vi "Global Data.vi"() -> ()   [LabVIEW 2014]
uses:
  BMS Telemetry.ctl
  Vehicle Status/Subsystem Status.ctl
  Vehicle Status/Subsystem Status Severity.ctl
  Vehicle Status/Subsystem Status Message.ctl
  FPGA Telemetry.ctl
  AIR Status.ctl
  Reason for Shutdown.ctl
  Dash LED Status.ctl
  FPGA/SPI v2/ADXL345 Output.ctl
  Shutdown State Machine.lvsc/State.ctl
  CAN/MC/MC Temp 1.ctl
  CAN/MC/MC Temp 2.ctl
  CAN/MC/MC Temp 3.ctl
  CAN/MC/MC Current.ctl
  CAN/MC/MC Voltage.ctl
  CAN/MC/MC State.ctl
  CAN/Inverter States.ctl
  CAN/Inverter Run Modes.ctl
  CAN/VSM States.ctl
  CAN/MC/MC Torque.ctl
  CAN/MC/MC Faults.ctl
  CAN/MC/MC Position.ctl
  MC State Machine.lvsc/State.ctl
  CAN/MC/MC Internal Voltages.ctl
  CAN/MC/MC Flux.ctl
  CAN/MC/MC Mod Index and Flux Weakening.ctl
  Dashboard/DashDriverInputs.ctl
  Lap Statistics.ctl
  Dashboard/SDashLEDs.ctl
  CAN/TX Library/CAN Message Queue.ctl
  CAN/TX Library/CAN Message.ctl
  Shutdown State Machine.lvsc
  MC State Machine.lvsc
panel:
  out "HighPriorityCANQueue":T1
  out "LowPriorityCANQueue":T1
  out "MPowerLimiterCorrection":dbl
  out "SDashLEDs":T2
  out "RS232 Error Out":errorcluster
  in  "MTorqueRequest":dbl
  out "SLapStatistics":T3
  out "rAverageThrottle":dbl
  out "tRequestMCControl":dbl
  out "SDashDriverInputs":T4
  out "bPrechargeFailed":bool
  out "Mod Index & Flux Weakening":T5
  out "CAN Interface":refnum<k20>
  out "MC Flux":T6
  out "MC Internal Voltages":T7
  out "iPhone LF Data":cluster{"Lat":dbl, "Long":dbl, "Speed":dbl}
  out "iPhone HF Data":T8
  out "eMCStateMachine":T9=enum."Disabled"
  out "bNewCANLog":bool
  out "bNewSlowFPGALog":bool
  out "bNewFastFPGALog":bool
  in  "CLogFilePrefix":string
  in  "eReasonForShutdown":T10
  in  "bDisableAIRs":bool
  in  "bDisableMC":bool
  out "bRemoteReturnToPits":bool
  out "MC Position":T11
  out "MC Faults":T12 {"MC RUN" format="%x"; "MC Post" format="%x"}
  out "MC Torque":T13
  out "MC State":T14
  out "MC Voltage":T18
  out "MC Current":T19
  out "MC Temp 3":T20
  out "MC Temp 2":T21
  out "MC Temp 1":T22
  in  "bStopCode":bool
  out "eAIRStatus":T23
  out "eShutdownStateMachine":T24=enum."TSMS Off"
  in  "FPGA Telemetry":T25={"CPU Load"={"Total (%)"=16.524459104265105, "Time Critical (%)"=0.0023081499865067385, "Timed Structures (%)"=0.0005419957749163527, "High (%)"=0.304724766613852, "Above Normal (%)"=6.671544042254672, "Normal (%)"=9.519195244591105, "Background (%)"=0.026144905044047956, "Idle (%)"=83.4755408957349, "ISR (%)"=0.0}, "SVehicleStatus"={"BMS Status"={"eStatusSeverity"=enum."Okay", "NValue"=0.0, "CMessage"=enum."ControllerTemperature", "bNotOK"=FALSE}, "MC Status"={"eStatusSeverity"=enum."Okay", "NValue"=0.0, "CMessage"=enum."ControllerTemperature", "bNotOK"=FALSE}, "Shutdown Status"={"eStatusSeverity"=enum."Return to Pits", "NValue"=0.0, "CMessage"=enum."ControllerTemperature", "bNotOK"=FALSE}, "sbRIO Status"={"eStatusSeverity"=enum."Okay", "NValue"=0.0, "CMessage"=enum."ControllerTemperature", "bNotOK"=FALSE}, "Vehicle Status"={"eStatusSeverity"=enum."Return to Pits", "NValue"=0.0, "CMessage"=enum."ControllerTemperature", "bNotOK"=FALSE}, "Shutdown State"=enum."TSMS Off", "AIR Status"=enum."On", "Remote Return to Pits"=TRUE, "Reason for Shutdown"=enum."Shutdown", "MC State Machine Status"=enum."Disabled"}, "iPhone HF Data"={"gXiPhone"=0.0, "gYiPhone"=0.0, "gZiPhone"=0.0, "nYawXiPhone"=0.0, "nYawYiPhone"=0.0, "nYawZiPhone"=0.0}, "iPhone LF Data"={"nLatiPhone"=0.0, "nLongiPhone"=0.0, "nGPSiPhone"=0.0}, "stop"=TRUE, "VSupplyOffset"=0.3359375, "VsbRIOSupply"=0.3803386688232422, "bFPGALED"=TRUE, "TSBRIO"=0.3482666015625, "rTPS2Unscaled"=0.999969482421875, "rTPS1Unscaled"=0.999969482421875, "bTPSConsistent"=TRUE, "bTPSInRange"=FALSE, "rThrottle"=-11.19873046875, "VTPS2"=0.0, "rTPS2"=1.744140625, "VTPS1"=7.0, "rTPS1"=0.0, "rTPS2Max"=0.27001953125, "rTPS2Min"=0.489990234375, "rTPS1Max"=0.6201171875, "rTPS1Min"=0.41015625, "bCoolantPumpEnable"=FALSE, "bRTDSEnable"=TRUE, "bTSMSInStatus"=FALSE, "bPosAIREnable"=TRUE, "bBMSOK"=FALSE, "bIMDOK"=FALSE, "bBSPDOK"=TRUE, "bSBRIOOK2"=TRUE, "bSBRIOOK1"=TRUE, "bTSMSOutStatus"=TRUE, "eGreenDash"=enum."Off", "eYellowDash"=enum."Off", "eRedDash"=enum."Off", "bMotorControllerEnable"=TRUE, "tCurrentLap"=0, "bNewLap"=TRUE, "tLastLap"=0, "tLapMin"=0, "V5VSupply"=0.0, "bWheelRL"=TRUE, "bWheelRR"=TRUE, "bWheelFR"=FALSE, "bWheelFL"=FALSE, "VBrakePressureR"=0.4820976257324219, "VBrakePressureF"=0.4808177947998047, "bWheelRRStopped"=FALSE, "bWheelRLStopped"=FALSE, "bWheelFRStopped"=FALSE, "bWheelFLStopped"=TRUE, "tWheelRLPeriod"=0, "tWheelRRPeriod"=0, "tWheelFRPeriod"=0, "tWheelFLPeriod"=0, "bBrakeLight"=TRUE, "VShockRR"=0.3793773651123047, "VShockRL"=0.3444976806640625, "VShockFR"=0.3425788879394531, "VShockFL"=0.3892974853515625, "IHighCurrent"=-20.724609375, "ILowCurrent"=4.353515625, "pBrakeR"=0.0, "pBrakeF"=0.0, "bHighCurrentOK"=FALSE, "bLowCurrentOK"=FALSE, "bBrakeROK"=FALSE, "bBrakeFOK"=FALSE, "VSteerWheelMiddle"=0.34827280044555664, "aSteerWheel"=124.90449142456055, "nWheelFL"=0.0, "nWheelFR"=0.0, "nWheelRL"=0.0, "nWheelRR"=0.0, "ADXL345 Output"={"X"=0.0, "Y"=0.0, "Z"=0.0}, "Tire Diameter(m)"=0.0, "vWheelRR"=0.0, "vWheelRL"=0.0, "vWheelFR"=0.0, "vWheelFL"=0.0, "vWheelLowest"=0.0, "vWheelHighest"=0.0, "bAccel"=FALSE, "vAxleF"=0.0, "vCar"=0.0, "sLap"=0.0, "rSlipRL"=0.0, "rSlipRR"=0.0, "rSlipFL"=0.0, "rSlipFR"=0.0, "NLap"=0, "tLapReference"=0, "tFastestLap"=0, "MTorqueRequest"=0.0, "RS232 Error Out"={"status"=FALSE, "code"=0}} {"TSBRIO" format="%.10g"; "CPU Load"."ISR (%)" format="%#.2f"; "CPU Load"."Idle (%)" format="%#.2f"; "CPU Load"."Background (%)" format="%#.2f"; "CPU Load"."Normal (%)" format="%#.2f"; "CPU Load"."Above Normal (%)" format="%#.2f"; "CPU Load"."High (%)" format="%#.2g"; "CPU Load"."Time Critical (%)" format="%#.2g"}
  in  "SVehicleStatus":T26
  in  "SSBRIOStatus":T26
  in  "SShutdownStatus":T26
  in  "SMCStatus":T26
  in  "SBMSStatus":T26
  out "BMS Telemetry":T31={"bBMSIgnition"=FALSE, "bBMSChargerMains"=FALSE, "bBMSFastCharge"=FALSE, "bBMSChargerEnabled"=FALSE, "eBMSCarState"=enum."Off", "eBMSChargingState"=enum."Disconnected", "tBMSChargeStage"=32, "eBMSLastChargeError"=enum."No Error", "NBMSNumCells"=70, "bBMSUnderVProtection"=FALSE, "bBMSOverVProtection"=FALSE, "bBMSOverTProtection"=FALSE, "bBMSLeakageProtection"=FALSE, "bBMSNoCellCommsError"=FALSE, "bBMSLowVReduction"=FALSE, "bBMSHighTReduction"=FALSE, "VCellMin"=3.84, "VCellMax"=4.2, "VCellMean"=4.0600000000000005, "VTotal"=284.33, "TCellMin"=17.0, "TCellMax"=43.0, "TCellMean"=20.0, "VCells"={"[51]"=4.08, "[52]"=4.05, "[53]"=4.1, "[54]"=4.2, "[55]"=0.0, "[56]"=4.109999999999999, "[57]"=4.1, "[58]"=4.1899999999999995, "[59]"=4.109999999999999, "[60]"=4.07, "[61]"=4.1, "[62]"=4.220000000000001, "[63]"=0.0, "[64]"=4.07, "[65]"=4.05, "[66]"=4.109999999999999, "[67]"=4.12, "[34]"=3.95, "[35]"=4.05, "[36]"=4.1, "[37]"=4.08, "[38]"=4.05, "[39]"=0.0, "[40]"=4.07, "[41]"=4.029999999999999, "[42]"=4.02, "[43]"=4.02, "[44]"=3.99, "[45]"=4.05, "[46]"=4.029999999999999, "[47]"=0.0, "[48]"=3.99, "[49]"=4.01, "[50]"=4.02, "[17]"=3.84, "[18]"=4.0600000000000005, "[19]"=4.05, "[20]"=3.99, "[21]"=4.02, "[22]"=4.02, "[23]"=0.0, "[24]"=4.07, "[25]"=4.01, "[26]"=4.140000000000001, "[27]"=4.02, "[28]"=4.05, "[29]"=4.029999999999999, "[30]"=4.08, "[31]"=0.0, "[32]"=4.109999999999999, "[33]"=4.02, "[0]"=2.0, "[1]"=2.0, "[2]"=2.0, "[3]"=2.0, "[4]"=2.0, "[5]"=2.0, "[6]"=2.0, "[7]"=0.0, "[8]"=4.02, "[9]"=4.07, "[10]"=4.029999999999999, "[11]"=4.02, "[12]"=4.02, "[13]"=4.05, "[14]"=4.0600000000000005, "[15]"=0.0, "[16]"=4.2}, "TCells"={"[55]"=0.0, "[56]"=21.0, "[57]"=21.0, "[58]"=33.0, "[59]"=21.0, "[60]"=23.0, "[61]"=21.0, "[62]"=43.0, "[63]"=0.0, "[64]"=22.0, "[65]"=21.0, "[66]"=21.0, "[67]"=19.0, "[68]"=21.0, "[69]"=20.0, "[70]"=-100.0, "[17]"=19.0, "[38]"=21.0, "[39]"=0.0, "[40]"=19.0, "[41]"=21.0, "[42]"=21.0, "[43]"=21.0, "[44]"=19.0, "[45]"=21.0, "[46]"=20.0, "[47]"=0.0, "[48]"=20.0, "[49]"=19.0, "[50]"=19.0, "[51]"=19.0, "[52]"=19.0, "[53]"=19.0, "[54]"=33.0, "[21]"=20.0, "[22]"=20.0, "[23]"=0.0, "[24]"=21.0, "[25]"=21.0, "[26]"=21.0, "[27]"=19.0, "[28]"=19.0, "[29]"=19.0, "[30]"=19.0, "[31]"=0.0, "[32]"=19.0, "[33]"=19.0, "[34]"=19.0, "[35]"=19.0, "[36]"=19.0, "[37]"=19.0, "[0]"=19.0, "[1]"=17.0, "[2]"=19.0, "[3]"=19.0, "[4]"=19.0, "[5]"=19.0, "[6]"=19.0, "[7]"=0.0, "[8]"=21.0, "[9]"=19.0, "[10]"=20.0, "[11]"=19.0, "[12]"=21.0, "[13]"=19.0, "[14]"=19.0, "[15]"=0.0, "[16]"=25.0}, "bChargerConnected"=FALSE, "VChargerSetpoint"=0.0, "IChargerSetpoint"=0.0, "VChargerActual"=0.0, "IChargerActual"=0.0, "BCells"={"[51]"=0.0, "[52]"=0.0, "[53]"=0.0, "[54]"=0.0, "[55]"=0.0, "[56]"=0.0, "[57]"=0.0, "[58]"=0.0, "[59]"=0.0, "[60]"=0.0, "[61]"=0.0, "[62]"=0.0, "[63]"=0.0, "[64]"=0.0, "[65]"=0.0, "[66]"=0.0, "[67]"=0.0, "[34]"=0.0, "[35]"=0.0, "[36]"=0.0, "[37]"=0.0, "[38]"=0.0, "[39]"=0.0, "[40]"=0.0, "[41]"=0.0, "[42]"=0.0, "[43]"=0.0, "[44]"=0.0, "[45]"=0.0, "[46]"=0.0, "[47]"=0.0, "[48]"=0.0, "[49]"=0.0, "[50]"=0.0, "[17]"=0.0, "[18]"=0.0, "[19]"=0.0, "[20]"=0.0, "[21]"=0.0, "[22]"=0.0, "[23]"=0.0, "[24]"=0.0, "[25]"=0.0, "[26]"=0.0, "[27]"=0.0, "[28]"=0.0, "[29]"=0.0, "[30]"=0.0, "[31]"=0.0, "[32]"=0.0, "[33]"=0.0, "[0]"=0.0, "[1]"=0.0, "[2]"=0.0, "[3]"=0.0, "[4]"=0.0, "[5]"=0.0, "[6]"=0.0, "[7]"=0.0, "[8]"=0.0, "[9]"=0.0, "[10]"=0.0, "[11]"=0.0, "[12]"=0.0, "[13]"=0.0, "[14]"=0.0, "[15]"=0.0, "[16]"=0.0}}
  in  "bMCOn":bool
  in  "bEnableRTDS":bool
  in  "nHeading":i16
  in  "nChassis":dbl
  # "MC Telemetry"
  # "Inputs"
  # "Protection"
  # "State"
  # "Outputs"
  # "Reduction"
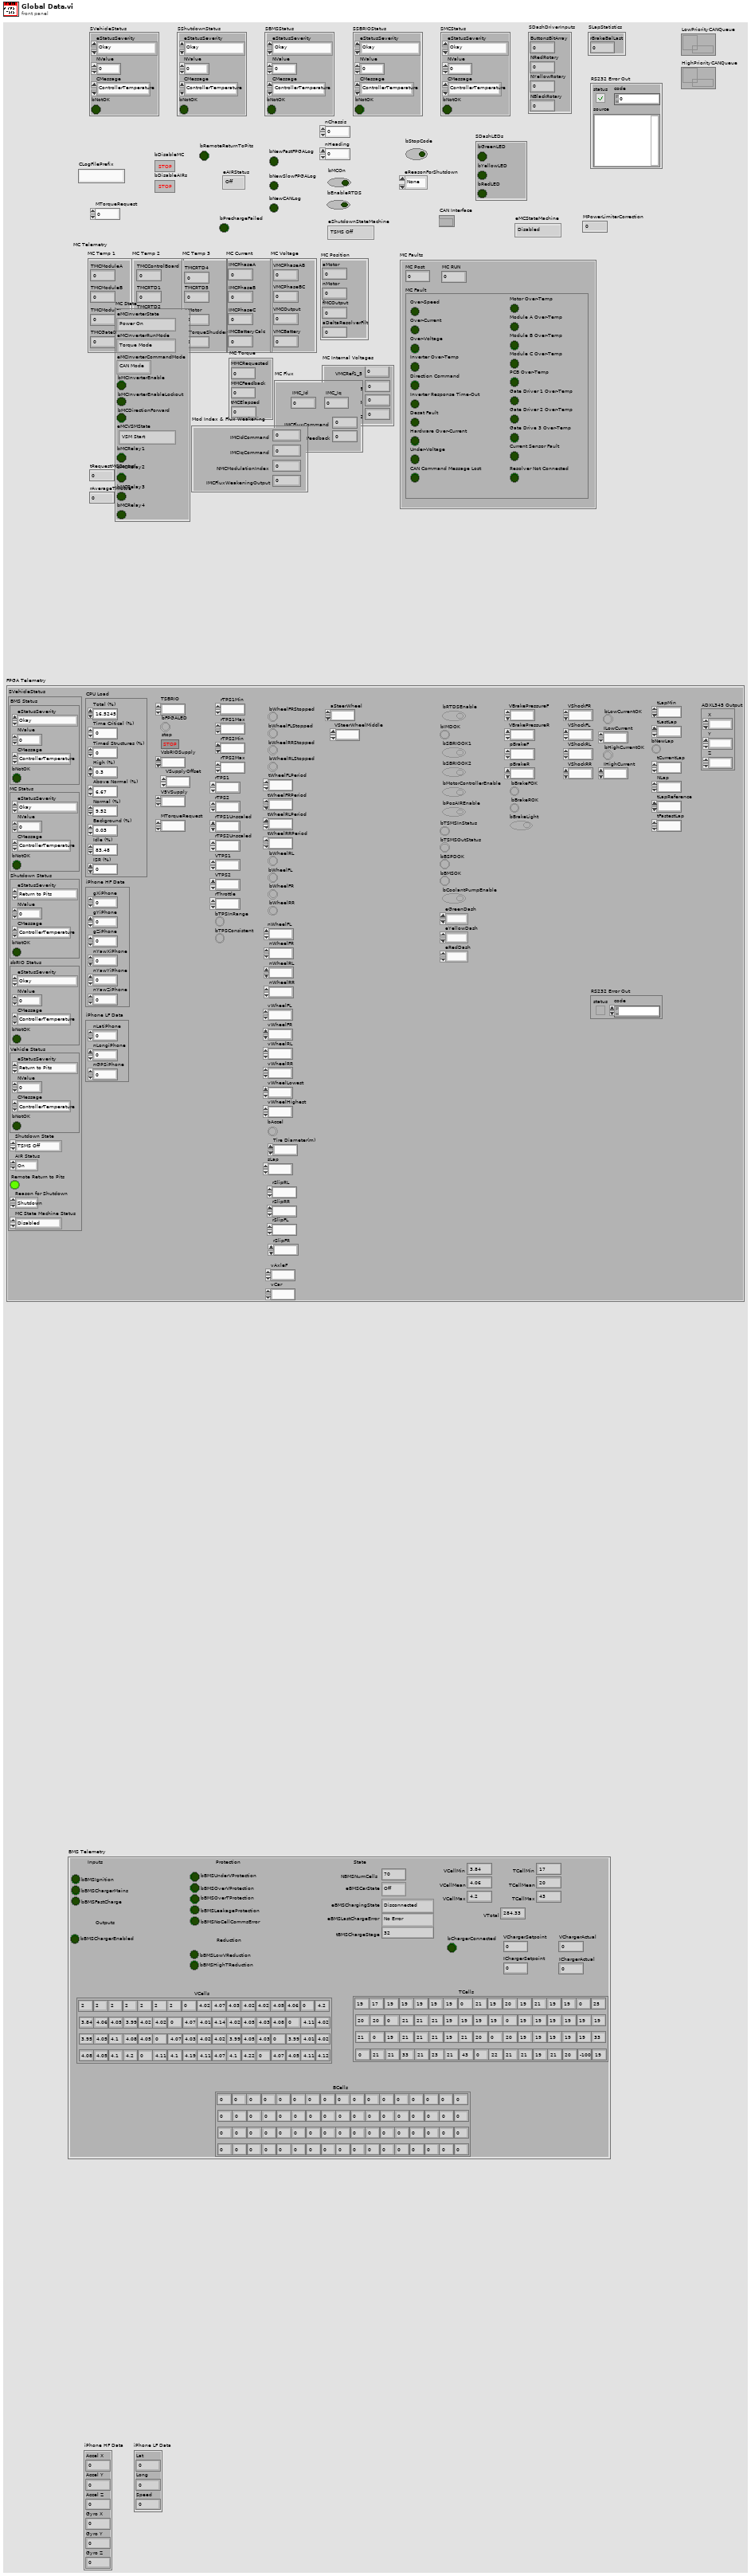
[diagram p1: front panel]
types:
  T1 = typedef "CAN Message Queue.ctl" = refnum<k33>
  T2 = typedef "SDashLEDs.ctl" = cluster{"bGreenLED":bool, "bYellowLED":bool, "bRedLED":bool}
  T3 = typedef "Lap Statistics.ctl" = cluster{"rBrakeBalLast":dbl}
  T4 = typedef "DashDriverInputs.ctl" = cluster{"ButtonsBitArray":u8, "NRedRotary":u8, "NYellowRotary":u8, "NBlackRotary":u8}
  T5 = typedef "MC Mod Index and Flux Weakening.ctl" = cluster{"NMCModulationIndex":dbl, "IMCFluxWeakeningOutput":dbl, "IMCIdCommand":dbl, "IMCIqCommand":dbl}
  T6 = typedef "MC Flux.ctl" = cluster{"IMCFluxCommand":dbl, "IMCFluxFeedback":dbl, "IMC_Id":dbl, "IMC_Iq":dbl}
  T7 = typedef "MC Internal Voltages.ctl" = cluster{"VMCRef1_5":dbl, "VMCRef2_5":dbl, "VMCRef5":dbl, "VMCRef12":dbl}
  T8 = cluster{"Accel X":dbl, "Accel Y":dbl, "Accel Z":dbl, "Gyro X":dbl, "Gyro Y":dbl, "Gyro Z":dbl}
  T9 = typedef "MC State Machine.lvsc/State.ctl" = enum16{"NI.SC.Initial", "NI.SC.History", "NI.SC.ShallowHistory", "NI.SC.Terminal", "Broadcast Diag", "Let Current Drop then Disable AIR's", "Enabled", "Disabled"}
  T10 = typedef "Reason for Shutdown.ctl" = enum16{"None", "BMS", "Shutdown", "sbRIO", "MC", "Remote"}
  T11 = typedef "MC Position.ctl" = cluster{"aMotor":dbl, "nMotor":dbl, "fMCOutput":dbl, "aDeltaResolverFilt":dbl}
  T12 = typedef "MC Faults.ctl" = cluster{"MC Fault":cluster{"Over-Speed":bool, "Over-Current":bool, "Over-Voltage":bool, "Inverter Over-Temp":bool, "Direction Command":bool, "Inverter Response Time-Out":bool, "Desat Fault":bool, "Hardware Over-Current":bool, "Under-Voltage":bool, "CAN Command Message Lost":bool, "Motor Over-Temp":bool, "Module A Over-Temp":bool, "Module B Over-Temp":bool, "Module C Over-Temp":bool, "PCB Over-Temp":bool, "Gate Driver 1 Over-Temp":bool, "Gate Driver 2 Over-Temp":bool, "Gate Drive 3 Over-Temp":bool, "Current Sensor Fault":bool, "Resolver Not Connected":bool}, "MC Post":u32, "MC RUN":u32}
  T13 = typedef "MC Torque.ctl" = cluster{"MMCRequested":dbl, "MMCFeedback":dbl, "tMCElapsed":u32}
  T14 = typedef "MC State.ctl" = cluster{"eMCInverterState":T15, "eMCInverterRunMode":T16, "eMCInverterCommandMode":enum16{"CAN Mode", "VSM Mode"}, "bMCInverterEnable":bool, "bMCInverterEnableLockout":bool, "bMCDirectionForward":bool, "eMCVSMState":T17, "bMCRelay1":bool, "bMCRelay2":bool, "bMCRelay3":bool, "bMCRelay4":bool}
  T15 = typedef "Inverter States.ctl" = enum16{"Power On", "Stop", "Open Loop", "Closed Loop", "Wait", "Internal", "Idle Run", "Idle Stop", ""}
  T16 = typedef "Inverter Run Modes.ctl" = enum16{"Torque Mode", "Speed Mode"}
  T17 = typedef "VSM States.ctl" = enum16{"VSM Start", "Pre-Charge Init", "Pre-Charge Active", "Pre-Charge Complete", "VSM Wait", "VSM Ready", "Motor Running", "Blink Fault Code", "Shutdown in Process", "Recycle Power"}
  T18 = typedef "MC Voltage.ctl" = cluster{"VMCPhaseAB":dbl, "VMCPhaseBC":dbl, "VMCOutput":dbl, "VMCBattery":dbl}
  T19 = typedef "MC Current.ctl" = cluster{"IMCPhaseA":dbl, "IMCPhaseB":dbl, "IMCPhaseC":dbl, "IMCBatteryCalc":dbl}
  T20 = typedef "MC Temp 3.ctl" = cluster{"TMCRTD4":dbl, "TMCRTD5":dbl, "TMotor":dbl, "MTorqueShudder":dbl}
  T21 = typedef "MC Temp 2.ctl" = cluster{"TMCControlBoard":dbl, "TMCRTD1":dbl, "TMCRTD2":dbl, "TMCRTD3":dbl}
  T22 = typedef "MC Temp 1.ctl" = cluster{"TMCModuleA":dbl, "TMCModuleB":dbl, "TMCModuleC":dbl, "TMCGateDriver":dbl}
  T23 = typedef "AIR Status.ctl" = enum16{"Off", "Precharge", "On"}
  T24 = typedef "Shutdown State Machine.lvsc/State.ctl" = enum16{"NI.SC.Initial", "NI.SC.History", "NI.SC.ShallowHistory", "NI.SC.Terminal", "Coolant Pump Started/AIR's On", "AIRs On", "Precharge", "TSMS Off"}
  T25 = typedef "FPGA Telemetry.ctl" = cluster{"CPU Load":cluster{"Total (%)":dbl, "Time Critical (%)":dbl, "Timed Structures (%)":dbl, "High (%)":dbl, "Above Normal (%)":dbl, "Normal (%)":dbl, "Background (%)":dbl, "Idle (%)":dbl, "ISR (%)":dbl}, "SVehicleStatus":cluster{"BMS Status":T26, "MC Status":T26, "Shutdown Status":T26, "sbRIO Status":T26, "Vehicle Status":T26, "Shutdown State":enum16{"NI.SC.Initial", "NI.SC.History", "NI.SC.ShallowHistory", "NI.SC.Terminal", "Coolant Pump Started/AIR's On", "AIRs On", "Precharge", "TSMS Off"}, "AIR Status":T23, "Remote Return to Pits":bool, "Reason for Shutdown":T10, "MC State Machine Status":enum16{"NI.SC.Initial", "NI.SC.History", "NI.SC.ShallowHistory", "NI.SC.Terminal", "Broadcast Diag", "Let Current Drop then Disable AIR's", "Enabled", "Disabled"}}, "iPhone HF Data":cluster{"gXiPhone":dbl, "gYiPhone":dbl, "gZiPhone":dbl, "nYawXiPhone":dbl, "nYawYiPhone":dbl, "nYawZiPhone":dbl}, "iPhone LF Data":cluster{"nLatiPhone":dbl, "nLongiPhone":dbl, "nGPSiPhone":dbl}, "stop":bool, "VSupplyOffset":fxp<+,12,4>, "VsbRIOSupply":fxp<+/-,25,6>, "bFPGALED":bool, "TSBRIO":fxp<+/-,33,17>, "rTPS2Unscaled":fxp<+/-,16,1>, "rTPS1Unscaled":fxp<+/-,16,1>, "bTPSConsistent":bool, "bTPSInRange":bool, "rThrottle":fxp<+/-,33,22>, "VTPS2":fxp<+/-,24,5>, "rTPS2":fxp<+/-,31,22>, "VTPS1":fxp<+/-,24,5>, "rTPS1":fxp<+/-,31,22>, "rTPS2Max":fxp<+,16,4>, "rTPS2Min":fxp<+,16,4>, "rTPS1Max":fxp<+,16,4>, "rTPS1Min":fxp<+,16,4>, "bCoolantPumpEnable":bool, "bRTDSEnable":bool, "bTSMSInStatus":bool, "bPosAIREnable":bool, "bBMSOK":bool, "bIMDOK":bool, "bBSPDOK":bool, "bSBRIOOK2":bool, "bSBRIOOK1":bool, "bTSMSOutStatus":bool, "eGreenDash":T29, "eYellowDash":T29, "eRedDash":T29, "bMotorControllerEnable":bool, "tCurrentLap":u32, "bNewLap":bool, "tLastLap":u32, "tLapMin":u32, "V5VSupply":fxp<+/-,24,5>, "bWheelRL":bool, "bWheelRR":bool, "bWheelFR":bool, "bWheelFL":bool, "VBrakePressureR":fxp<+/-,24,5>, "VBrakePressureF":fxp<+/-,24,5>, "bWheelRRStopped":bool, "bWheelRLStopped":bool, "bWheelFRStopped":bool, "bWheelFLStopped":bool, "tWheelRLPeriod":u32, "tWheelRRPeriod":u32, "tWheelFRPeriod":u32, "tWheelFLPeriod":u32, "bBrakeLight":bool, "VShockRR":fxp<+/-,24,5>, "VShockRL":fxp<+/-,24,5>, "VShockFR":fxp<+/-,24,5>, "VShockFL":fxp<+/-,24,5>, "IHighCurrent":fxp<+/-,24,15>, "ILowCurrent":fxp<+/-,24,15>, "pBrakeR":fxp<+,26,13>, "pBrakeF":fxp<+,26,13>, "bHighCurrentOK":bool, "bLowCurrentOK":bool, "bBrakeROK":bool, "bBrakeFOK":bool, "VSteerWheelMiddle":fxp<+/-,26,5>, "aSteerWheel":fxp<+/-,31,13>, "nWheelFL":fxp<+/-,32,16>, "nWheelFR":fxp<+/-,32,16>, "nWheelRL":fxp<+/-,32,16>, "nWheelRR":fxp<+/-,32,16>, "ADXL345 Output":T30, "Tire Diameter(m)":fxp<+,16,1>, "vWheelRR":fxp<+/-,32,18>, "vWheelRL":fxp<+/-,32,18>, "vWheelFR":fxp<+/-,32,18>, "vWheelFL":fxp<+/-,32,18>, "vWheelLowest":fxp<+/-,32,18>, "vWheelHighest":fxp<+/-,32,18>, "bAccel":bool, "vAxleF":fxp<+/-,33,19>, "vCar":fxp<+/-,33,19>, "sLap":fxp<+,32,12>, "rSlipRL":fxp<+/-,12,1>, "rSlipRR":fxp<+/-,12,1>, "rSlipFL":fxp<+/-,12,1>, "rSlipFR":fxp<+/-,12,1>, "NLap":u8, "tLapReference":u32, "tFastestLap":u32, "MTorqueRequest":dbl, "RS232 Error Out":cluster{"status":bool, "code":i32}}
  T26 = typedef "Subsystem Status.ctl" = cluster{"eStatusSeverity":T27, "NValue":sgl, "CMessage":T28, "bNotOK":bool}
  T27 = typedef "Subsystem Status Severity.ctl" = enum16{"Okay", "Short Warning", "Long Warning", "Return to Pits", "Error", "Danger"}
  T28 = typedef "Subsystem Status Message.ctl" = enum16{"ControllerTemperature", "MotorTemperature", "BatteryTemperature", "BatteryLowVoltage", "LVBattery", "sbRIOTemperature", "Precharge", "BSPD", "IMD", "RemoteReturnToPits", "EStopInterrupted", "NoCellComms", "MCOverSpeed", "MCOverCurrent", "MCOverVoltage", "MCInverterOverTemp", "MCDirectionCommand", "MCInverterTimeout", "MCDesatFault", "MCHWOverCurrent", "MCUnderVoltage", "MCCommandMessageLost", "MotorOverTemp", "MCModAOverTemp", "MCModBOverTemp", "MCModCOverTemp", "MCPCBOverTemp", "MCGateDrv1OverTemp", "MCDateDrv2OverTemp", "MCCurrentSensorFault", "MCResolverNotConnected", "ShutdownLatchTripped", "UnknownBMS", "RemoteEmergency"}
  T29 = typedef "Dash LED Status.ctl" = enum16{"Off", "Flashing", "On"}
  T30 = typedef "ADXL345 Output.ctl" = cluster{"X":fxp<+/-,14,4>, "Y":fxp<+/-,14,4>, "Z":fxp<+/-,14,4>}
  T31 = typedef "BMS Telemetry.ctl" = cluster{"bBMSIgnition":bool, "bBMSChargerMains":bool, "bBMSFastCharge":bool, "bBMSChargerEnabled":bool, "eBMSCarState":enum16{"Off", "On, Not Charging", "Charging", "Charging Finished", "Charging Error"}, "eBMSChargingState":enum16{"Disconnected", "Pre-charging", "Main Charging", "Balancing", "Charging Finished OK", "Charging Error"}, "tBMSChargeStage":u16, "eBMSLastChargeError":enum16{"No Error", "No Cell Communication", "No Cell Communication - Non CAN Charger", "Maximum charging stage duration expired", "Cell Communication Lost during Charge", "Cannot set balancing voltage", "Cell temps too high", "No Comms so can't determine temp", "# of Cells Mismatch", "Cells Overvoltage", "Cell Protection Event occured."}, "NBMSNumCells":u8, "bBMSUnderVProtection":bool, "bBMSOverVProtection":bool, "bBMSOverTProtection":bool, "bBMSLeakageProtection":bool, "bBMSNoCellCommsError":bool, "bBMSLowVReduction":bool, "bBMSHighTReduction":bool, "VCellMin":dbl, "VCellMax":dbl, "VCellMean":dbl, "VTotal":dbl, "TCellMin":dbl, "TCellMax":dbl, "TCellMean":dbl, "VCells":cluster{"[51]":dbl, "[52]":dbl, "[53]":dbl, "[54]":dbl, "[55]":dbl, "[56]":dbl, "[57]":dbl, "[58]":dbl, "[59]":dbl, "[60]":dbl, "[61]":dbl, "[62]":dbl, "[63]":dbl, "[64]":dbl, "[65]":dbl, "[66]":dbl, "[67]":dbl, "[34]":dbl, "[35]":dbl, "[36]":dbl, "[37]":dbl, "[38]":dbl, "[39]":dbl, "[40]":dbl, "[41]":dbl, "[42]":dbl, "[43]":dbl, "[44]":dbl, "[45]":dbl, "[46]":dbl, "[47]":dbl, "[48]":dbl, "[49]":dbl, "[50]":dbl, "[17]":dbl, "[18]":dbl, "[19]":dbl, "[20]":dbl, "[21]":dbl, "[22]":dbl, "[23]":dbl, "[24]":dbl, "[25]":dbl, "[26]":dbl, "[27]":dbl, "[28]":dbl, "[29]":dbl, "[30]":dbl, "[31]":dbl, "[32]":dbl, "[33]":dbl, "[0]":dbl, "[1]":dbl, "[2]":dbl, "[3]":dbl, "[4]":dbl, "[5]":dbl, "[6]":dbl, "[7]":dbl, "[8]":dbl, "[9]":dbl, "[10]":dbl, "[11]":dbl, "[12]":dbl, "[13]":dbl, "[14]":dbl, "[15]":dbl, "[16]":dbl}, "TCells":cluster{"[55]":dbl, "[56]":dbl, "[57]":dbl, "[58]":dbl, "[59]":dbl, "[60]":dbl, "[61]":dbl, "[62]":dbl, "[63]":dbl, "[64]":dbl, "[65]":dbl, "[66]":dbl, "[67]":dbl, "[68]":dbl, "[69]":dbl, "[70]":dbl, "[17]":dbl, "[38]":dbl, "[39]":dbl, "[40]":dbl, "[41]":dbl, "[42]":dbl, "[43]":dbl, "[44]":dbl, "[45]":dbl, "[46]":dbl, "[47]":dbl, "[48]":dbl, "[49]":dbl, "[50]":dbl, "[51]":dbl, "[52]":dbl, "[53]":dbl, "[54]":dbl, "[21]":dbl, "[22]":dbl, "[23]":dbl, "[24]":dbl, "[25]":dbl, "[26]":dbl, "[27]":dbl, "[28]":dbl, "[29]":dbl, "[30]":dbl, "[31]":dbl, "[32]":dbl, "[33]":dbl, "[34]":dbl, "[35]":dbl, "[36]":dbl, "[37]":dbl, "[0]":dbl, "[1]":dbl, "[2]":dbl, "[3]":dbl, "[4]":dbl, "[5]":dbl, "[6]":dbl, "[7]":dbl, "[8]":dbl, "[9]":dbl, "[10]":dbl, "[11]":dbl, "[12]":dbl, "[13]":dbl, "[14]":dbl, "[15]":dbl, "[16]":dbl}, "bChargerConnected":bool, "VChargerSetpoint":dbl, "IChargerSetpoint":dbl, "VChargerActual":dbl, "IChargerActual":dbl, "BCells":cluster{"[51]":dbl, "[52]":dbl, "[53]":dbl, "[54]":dbl, "[55]":dbl, "[56]":dbl, "[57]":dbl, "[58]":dbl, "[59]":dbl, "[60]":dbl, "[61]":dbl, "[62]":dbl, "[63]":dbl, "[64]":dbl, "[65]":dbl, "[66]":dbl, "[67]":dbl, "[34]":dbl, "[35]":dbl, "[36]":dbl, "[37]":dbl, "[38]":dbl, "[39]":dbl, "[40]":dbl, "[41]":dbl, "[42]":dbl, "[43]":dbl, "[44]":dbl, "[45]":dbl, "[46]":dbl, "[47]":dbl, "[48]":dbl, "[49]":dbl, "[50]":dbl, "[17]":dbl, "[18]":dbl, "[19]":dbl, "[20]":dbl, "[21]":dbl, "[22]":dbl, "[23]":dbl, "[24]":dbl, "[25]":dbl, "[26]":dbl, "[27]":dbl, "[28]":dbl, "[29]":dbl, "[30]":dbl, "[31]":dbl, "[32]":dbl, "[33]":dbl, "[0]":dbl, "[1]":dbl, "[2]":dbl, "[3]":dbl, "[4]":dbl, "[5]":dbl, "[6]":dbl, "[7]":dbl, "[8]":dbl, "[9]":dbl, "[10]":dbl, "[11]":dbl, "[12]":dbl, "[13]":dbl, "[14]":dbl, "[15]":dbl, "[16]":dbl}}
diagram:
